vi "Read File.vi"() -> (0 "Objects":T1(array[cluster]) {"Aspect Ratio" format="%.2f"; "Orientation" format="%.2f"; "Area" format="%.2f"; "Object Center"."Y" format="%.2f"; "Object Center"."X" format="%.2f"}, 2 "Total Obj":i32)   [LabVIEW 2012]
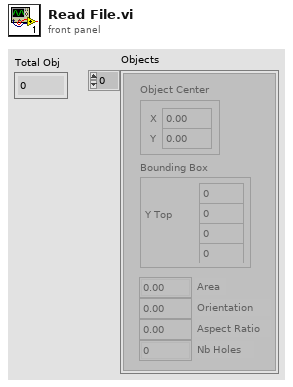
[diagram p1: front panel]
types:
  T1 = cluster{"Object Center":cluster{"X":sgl, "Y":sgl}, "Bounding Box":cluster{"X Left":i32, "Y Top":i32, "X Right":i32, "Y Bottom":i32}, "Area":sgl, "Orientation":sgl, "Aspect Ratio":sgl, "Nb Holes":i32}[]
  T2 = cluster{cluster{dbl, dbl}, cluster{i32, i32, i32, i32}, i32, i32, i32, i32}
  T3 = cluster{cluster{dbl, dbl}, cluster{i32, i32, i32, i32}, i32, i32, i32, i32}[]
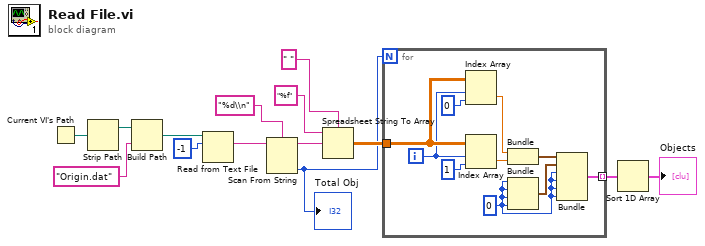
[diagram p0: block diagram]
diagram:
  n1 = Current VI's Path() -> (path=w6:path)
  n2 = Strip Path(path=w6) -> (stripped path=w8:path)  [unwired: 1 out]
  n3 = Build Path(base path=w8, name or relative path="Origin.dat" ("standard input")) -> (appended path=w5:path)
  n4 = Read from Text File(file (use dialog)=w5, count=-1) -> (text=w4:string)  [unwired: 2 in, 3 out]
  n5 = Scan From String(format string="%d\\n", input string=w4) -> (remaining string=w13:string, output 1=w3:i32)  [unwired: 3 in, 2 out]
  "Total Obj" <- w3
  n6 = Spreadsheet String To Array(delimiter (Tab)=" ", format string="%f", spreadsheet string=w13) -> (array=w10:dbl[][])  [unwired: 1 in]
  n7 = for {
    N: w3 -> [_]
    tunnel: [w21] -> w2 mode=indexing
    tunnel: w10 -> [w18]
    i -> [w17]
    w23 = 0
    n8 = Index Array(array=w18, index (row)=w17, index (col)=0) -> (element=w19:dbl)
    n9 = Index Array(array=w18, index (row)=w17, index (col)=1) -> (element=w15:dbl)
    n10 = Bundle(w19, w15) -> (w24:cluster{dbl, dbl})  [unwired: 1 in]
    n11 = Bundle(w23, w23, w23, w23) -> (w22:cluster{i32, i32, i32, i32})  [unwired: 1 in]
    n12 = Bundle(w24, w22, w23, w23, w23, w23) -> (w21:T2)  [unwired: 1 out]
  }
  n13 = Sort 1D Array(array=w2) -> (sorted array=→"Objects":T3)
